vi "Front Panel.vi"(11 "GUI In":refnum<class "PAS HF UI.lvclass">) -> ()   [LabVIEW 2015, in "PAS HF UI.lvclass"]
uses:
  PAS HF UI.lvclass
  Reusable/GUI/GUI.lvclass/GUI.ctl
  Reusable/Observer/Observer.lvclass/Observer.ctl
  Data/cPAS Data.lvclass
  Reusable/GUI/Accessors/Read RegEvent.vi
  Reusable/Observer/Read Data Queue.vi
  Reusable/PAS/Data/Main/Read CellData.vi
  Reusable/Data/Read measTime.vi
  Reusable/PAS/Data/Main/Read drive.vi
  Reusable/PAS/Data/Cell/Read timeData.vi
  Reusable/PAS/Data/Cell/Read lasDiodeData.vi
  Reusable/PAS/Data/Cell/Read Fitted Data.vi
  Reusable/PAS/Data/Cell/Read freqData.vi
  Reusable/PAS/Data/Cell/Read f0.vi
  Reusable/PAS/Data/Cell/Read Q.vi
  Reusable/Data/Data.lvclass
  Reusable/PAS/Data/Cell/PAS Cell Data.lvclass
panel:
  in  "f_cent":i16 caption="Center \nFrequency (Hz)"
  in  "Df":i16 caption="Bandwidth (Hz)"
  in  "log_lin":bool
  out "Q":sgl format="%.2f"
  out "f0":sgl
  in  "cell":T1(ring)
  out "micTime":waveform(i16)(graph) caption="Time Domain"
  out "micFreq":cluster{i32, dbl, "Y":sgl[]}[](graph) caption="Frequency Domain"
  out "diodeTime":waveform(i16)(graph) caption="Photodiode Time Domain"
  out "lastCal":timestamp caption="Last Speaker Calibration" format="%<%H:%M:%S>T"
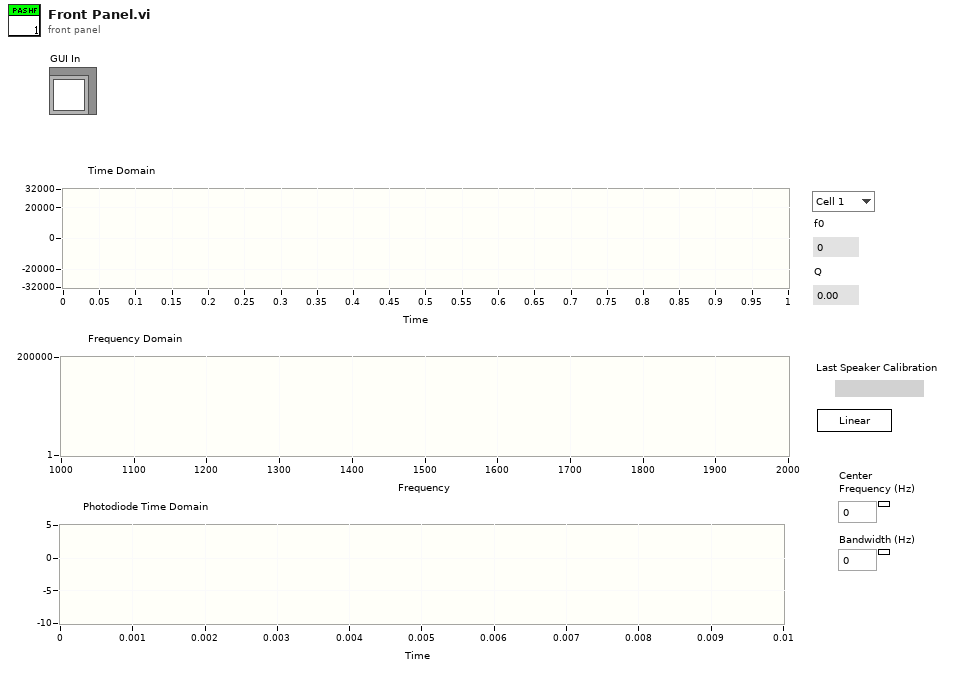
[diagram p1: front panel]
types:
  T1 = enum16{"Cell 1", "Cell 2", "Cell 3", "Cell 4", "Cell 5"}
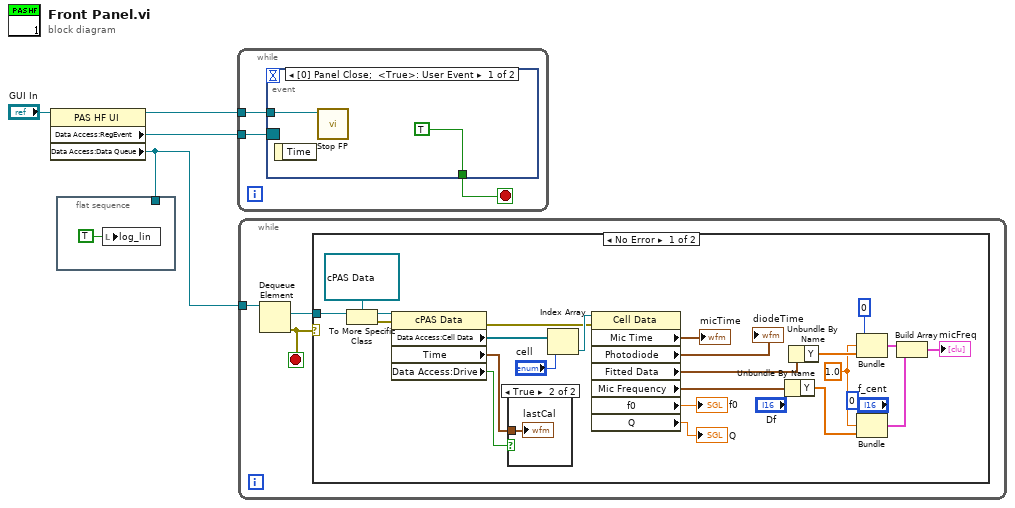
[diagram p0: block diagram]
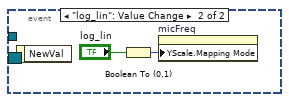
[diagram p2: hidden frame]
diagram:
  n1 = property class="PAS HF UI"(reference="GUI In") -> (reference out=w2:refnum<class "PAS HF UI.lvclass">, "Data Access:RegEvent"=w3:refnum<event-registration>, "Data Access:Data Queue"=w1:refnum<queue>)  [unwired: 1 in, 1 out]
  n2 = flat-sequence {
    tunnel: w1 -> [_]
    frame #0 {
      n3 = local write "log_lin"(TRUE ("log_lin")) -> ()
    }
  }
  n4 = while {
    tunnel: w3 -> [w7]
    tunnel: w2 -> [w6]
    stop <- w8 stop-if-true
    n5 = event shown="[0] Panel Close;  <True>: User Event" {
      selector: w7 -> [_ _]
      dyn-events: _ -> [_ _]
      timeout: _ -> [_ _]
      tunnel: [TRUE _] -> w8
      tunnel: w6 -> [w9 _]
      event Panel Close; User Event {
        n6 = event-data() -> ()  [unwired: 1 in, 1 out]
        n7 = call-dynamic "Stop FP.vi"("GUI in"=w9) -> ()  [unwired: 9 in, 2 out]
      }
      event "log_lin": Value Change {
        n8 = event-data() -> ()  [unwired: 1 in, 1 out]
        n9 = Boolean To (0,1)(Boolean="log_lin") -> (0, 1=w11:i16)
        n10 = property on="micFreq" class="WFGraph (strict)"("YScale.Mapping Mode"=w11) -> ()  [unwired: 2 in, 2 out]
      }
    }
  }
  n11 = while {
    tunnel: w1 -> [w15]
    stop <- w14 stop-if-true
    n12 = Dequeue Element(queue=w15) -> (element=w13:refnum<data-value>, error out=w14:errorcluster)  [unwired: 2 in, 2 out]
    n13 = case shown="No Error" w14 {
      tunnel: w13 -> [w21 _]
      frame No Error {
        w33 = 1.0
        n14 = To More Specific Class(target class=refnum<data-value> refnum ("data value reference"), reference=w21) -> (specific class reference=w20:refnum<data-value>, error out=w18:errorcluster)  [unwired: 1 in]
        n15 = property class="cPAS Data"(reference=w20, error in=w18) -> (error out=w36:errorcluster, "Data Access:Cell Data"=w39:refnum<class "PAS Cell Data.lvclass">[], "Time"=w16:timestamp, "Data Access:Drive"=w17:bool)  [unwired: 1 out]
        n16 = case shown="True" w17 {
          tunnel: w16 -> [_ w40]
          frame False {
          }
          frame True {
            "lastCal" <- w40
          }
        }
        n17 = Index Array(array=w39, index="cell") -> (element=w37:refnum<class "PAS Cell Data.lvclass">)
        n18 = property class="Cell Data"(reference=w37, error in=w36) -> ("Mic Time"=→"micTime":waveform(i16), "Photodiode"=→"diodeTime":waveform(i16), "Fitted Data"=w28:waveform(sgl), "Mic Frequency"=w27:waveform(sgl), "f0"=→"f0":sgl, "Q"=→"Q":sgl)  [unwired: 2 out]
        n19 = Unbundle By Name(w27) -> ("Y"=w35:sgl[])
        n20 = Unbundle By Name(w28) -> ("Y"=w34:sgl[])
        n21 = Bundle(0, w33, "Y"=w34) -> (w31:cluster{i32, dbl, "Y":sgl[]})  [unwired: 1 in]
        n22 = Bundle(0, w33, "Y"=w35) -> (w30:cluster{i32, dbl, "Y":sgl[]})  [unwired: 1 in]
        n23 = Build Array(w31, w30) -> (→"micFreq":cluster{i32, dbl, "Y":sgl[]}[])
      }
      frame Error {
      }
    }
  }
